vi "Actor Core.vi"(8 "error in":errorcluster, 11 "CS++DeviceGUIActor.lvclass":refnum<class "CS++DeviceGUIActor.lvclass">) -> (0 "Error Out":errorcluster, 3 "Actor out":refnum<class "Actor.lvclass">)   [LabVIEW 2014, in "CS++DeviceGUIActor.lvlib" / "CS++DeviceGUIActor.lvclass"]
doc: "(<B>Filename</B>: Actor Framework.lvlib:Actor.lvclass:Actor Core.vi)\n\nReceives messages to the actor, reacts to them, and initiates any error handling that may shut the actor down.\n\nDescendant classes may override this VI to append parallel tasks for the actor to complete while it handles messages. Overrides use the Call Parent Method node."
uses:
  CS++DeviceGUIActor.lvclass
  <vilib>/ActorFramework/Actor/Actor.lvclass
  CS++BaseActor/CS++BaseActor.lvclass/CS++BaseActor.ctl
  <vilib>/ActorFramework/Actor/Actor.lvclass/Actor.ctl
  <vilib>/ActorFramework/Message Enqueuer/Message Enqueuer.lvclass/Message Enqueuer.ctl
  CS++SVMonitor/CS++SVMonitor.lvclass
  Classes/CS++ProcessVariables/ProcessVariable/PV.lvclass
  CS++DeviceGUIActor Messages/Update PV.lvclass
  CS++PVMonitor Messages/Register PVs Msg/Register PVs Msg.lvclass/Register PVs Msg.ctl
  CS++DeviceGUIActor.lvclass/CS++DeviceGUIActor.ctl
  CS++GUIActor/CS++GUIActor.lvclass/CS++GUIActor.ctl
  Classes/CS++ProcessVariables/ProcessVariable/PV.lvclass/PV.ctl
  Classes/CS++ProcessVariables/ProcessVariable/Read Data.vi
  Classes/CS++ProcessVariables/ProcessVariable/Read Name.vi
  Classes/CS++ProcessVariables/ProcessVariable/Read Timestamp.vi
  <vilib>/ActorFramework/Message Enqueuer/Init from Existing Queue.vi
  <vilib>/ActorFramework/Message Enqueuer/Enqueue.vi
  <vilib>/ActorFramework/Message Priority Queue/Priority Enqueue.vi
  <vilib>/ActorFramework/Stop Msg/Stop Msg.lvclass
  <vilib>/ActorFramework/Message Enqueuer/Message Enqueuer.lvclass
  CS++PVMonitor Messages/Register PVs Msg/Register PVs Msg.lvclass
  Classes/CS++BaseClasses/Factory/CS++Factory.lvclass
  CS++GUIActor/CS++GUIActor.lvclass
  CS++BaseActor/CS++BaseActor.lvclass
panel:
  out "Timestamp":timestamp
  out "Resource Name":string
  out "Self-Test Result Message":string
  out "Self-Test Result Code":i32
  out "Firmware Revision":string
  out "Driver Revision":string
  in  "Stop Button":bool
  out "Associated Actor":string
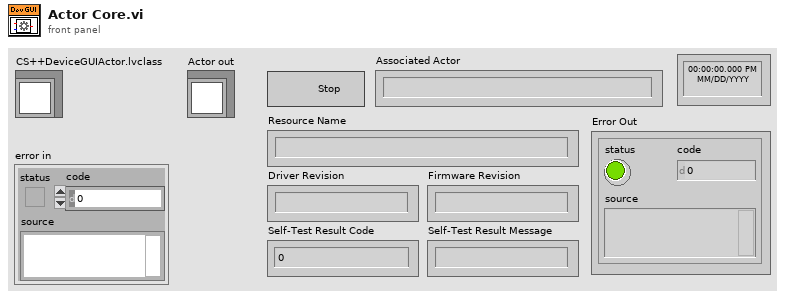
[diagram p1: front panel]
types:
  T1 = enum32{"Invalid", "Standard", "Closed", "Hidden", "Minimized", "Maximized"}
  T2 = cluster{string, "CS++DeviceGUIActor.lvlib:Update PV.lvclass":refnum<class "Update PV.lvclass">}
  T3 = cluster{"Self Enqueuer":refnum<class "Message Enqueuer.lvclass">, cluster{string, "CS++DeviceGUIActor.lvlib:Update PV.lvclass":refnum<class "Update PV.lvclass">}[]}
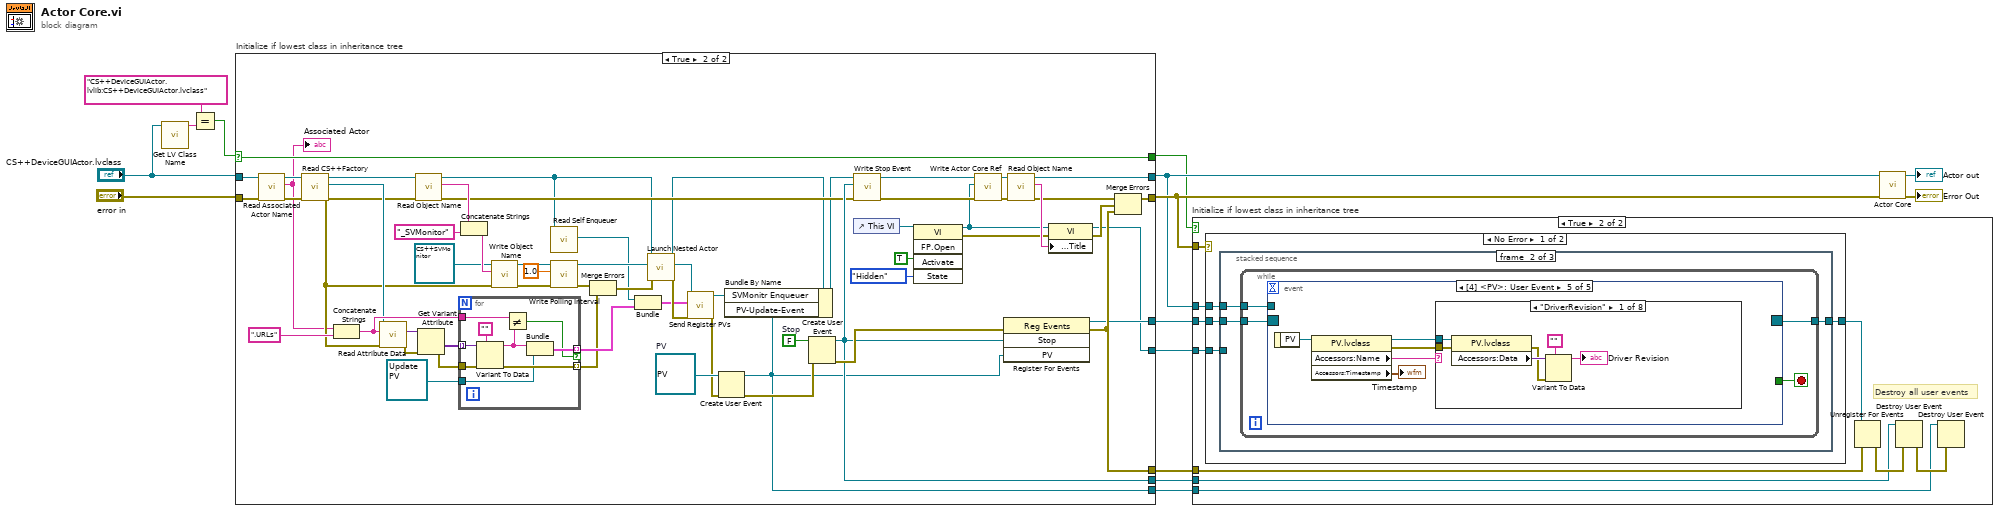
[diagram p0: block diagram]
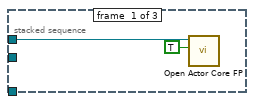
[diagram p4: hidden frame]
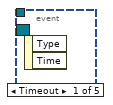
[diagram p5: hidden frame]
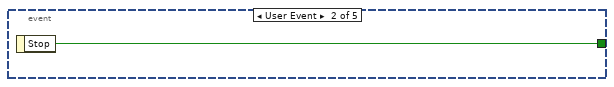
[diagram p6: hidden frame]
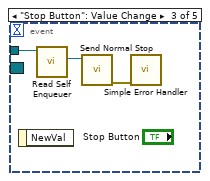
[diagram p7: hidden frame]
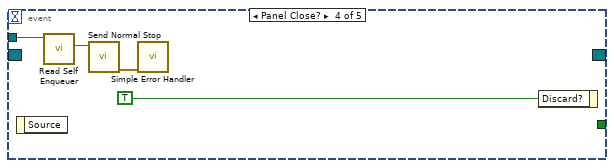
[diagram p8: hidden frame]
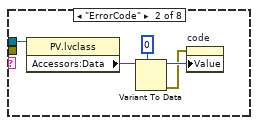
[diagram p9: hidden frame]
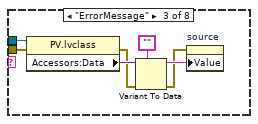
[diagram p10: hidden frame]
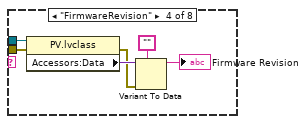
[diagram p11: hidden frame]
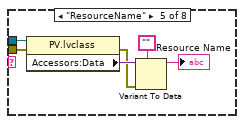
[diagram p12: hidden frame]
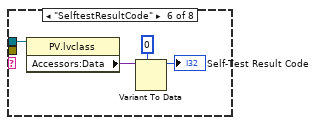
[diagram p13: hidden frame]
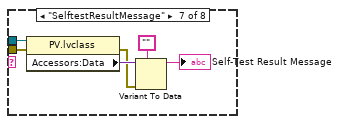
[diagram p14: hidden frame]
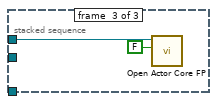
[diagram p16: hidden frame]
diagram:
  n1 = call <vilib>:"Get LV Class Name.vi"("object"="CS++DeviceGUIActor.lvclass") -> ("class name"=w9:string)  [unwired: 9 in, 1 out]
  n2 = Equal?(x="CS++DeviceGUIActor.lvlib:CS++DeviceGUIActor.lvclass" ("class name"), y=w9) -> (x = y?=w3:bool)
  n3 = case "Initialize if lowest class in inheritance tree" shown="True" w3 {
    selector: w3 -> [w16 w61]
    tunnel: [w17 w79] -> w13
    tunnel: "error in" -> [w17 w36]
    tunnel: [w18 w78] -> w11
    tunnel: "CS++DeviceGUIActor.lvclass" -> [w18 w35]
    tunnel: [_ w70] -> w7
    tunnel: [_ w69] -> w6
    tunnel: [_ w59] -> w5
    tunnel: [_ w67] -> w4
    tunnel: [w16 w61] -> w2
    tunnel: [_ w22] -> w1
    frame False {
    }
    frame True {
      w29 = refnum<class "PV.lvclass"> refnum  # PV
      w73 = FALSE  # Stop
      n4 = call "Read Associated Actor Name.vi"("error in (no error)"=w36, "CS++GUIActor in"=w35) -> ("error out"=w34:errorcluster, "Associated Actor Name"=w27:string, "CS++GUIActor out"=w33:refnum<class "CS++DeviceGUIActor.lvclass">)  [unwired: 7 in]
      "Associated Actor" <- w27
      n5 = call "Read CS++Factory.vi"("error in (no error)"=w34, "CS++BaseActor in"=w33) -> ("error out"=w30:errorcluster, "CS++Factory"=w32:refnum<class "CS++Factory.lvclass">, "CS++BaseActor out"=w31:refnum<class "CS++DeviceGUIActor.lvclass">)  [unwired: 7 in]
      n6 = Concatenate Strings(w27, ".URLs" ("string")) -> (w51:string)
      n7 = call-dynamic "Read Attribute Data.vi"("error in (no error)"=w30, "Object Name"=w51, "CS++Factory in"=w32) -> ("error out"=w57:errorcluster, "Attribute Data"=w56:variant)  [unwired: 6 in, 1 out]
      n8 = call "Read Object Name.vi"("error in (no error)"=w30, "CS++BaseActor in"=w31) -> ("error out"=w26:errorcluster, "Object Name"=w44:string, "CS++BaseActor out"=w20:refnum<class "CS++DeviceGUIActor.lvclass">)  [unwired: 7 in]
      n9 = Get Variant Attribute(Variant=w56, error in=w57) -> (values=w50:variant[], error out=w49:errorcluster)  [unwired: 2 in, 2 out]
      n10 = for {
        tunnel: [w88] -> w55 mode=indexing if=w84
        tunnel: w50 -> [w87] mode=indexing
        tunnel: w49 -> [w86]
        tunnel: w51 -> [w85]
        tunnel: [w81] -> w54 mode=indexing
        tunnel: refnum<class "Update PV.lvclass"> refnum ("CS++DeviceGUIActor.lvlib:Update PV.lvclass") -> [w80]
        n11 = Variant To Data(error in=w86, type="", Variant=w87) -> (data=w82:string, error out=w81:errorcluster)
        n12 = Not Equal?(x=w85, y=w82) -> (x != y?=w84:bool)
        n13 = Bundle(w82, "CS++DeviceGUIActor.lvlib:Update PV.lvclass"=w80) -> (w88:T2)  [unwired: 1 in]
      }
      n14 = Concatenate Strings(w44, "_SVMonitor" ("Object Name")) -> (w41:string)
      n15 = call "Write Object Name.vi"("error in (no error)"=w30, "Object Name"=w41, "CS++BaseActor in"=refnum<class "CS++SVMonitor.lvclass"> refnum ("CS++SVMonitor.lvlib:CS++SVMonitor.lvclass")) -> ("error out"=w38:errorcluster, "CS++BaseActor out"=w40:refnum<class "CS++SVMonitor.lvclass">)  [unwired: 7 in]
      n16 = call <vilib>:"Read Self Enqueuer.vi"("Actor"=w20) -> ("Self Enqueuer"=w45:refnum<class "Message Enqueuer.lvclass">)  [unwired: 10 in]
      n17 = call "Write Polling Interval.vi"("error in (no error)"=w38, "Polling Interval"=dbl[unit] 1.0 ("Interval"), "CS++BaseActor in"=w40) -> ("error out"=w52:errorcluster, "CS++BaseActor out"=w58:refnum<class "CS++SVMonitor.lvclass">)  [unwired: 7 in]
      n18 = Merge Errors(w52, w54) -> (w53:errorcluster)
      n19 = Bundle("Self Enqueuer"=w45, w55) -> (w46:T3)  [unwired: 1 in]
      n20 = call <vilib>:"Launch Nested Actor.vi"("error in (no error)"=w53, "Nested Actor"=w58, "Caller Actor in"=w20) -> ("error out"=w47:errorcluster, "Nested Actor's Enqueuer"=w37:refnum<class "Message Enqueuer.lvclass">, "Caller Actor out"=w19:refnum<class "CS++DeviceGUIActor.lvclass">)  [unwired: 6 in]
      n21 = call "Send Register PVs.vi"("error in (no error)"=w47, "Register Info"=w46, "Message Enqueuer"=w37) -> ("error out"=w25:errorcluster, "Message Enqueuer out"=w23:refnum<class "Message Enqueuer.lvclass">)  [unwired: 7 in]
      n22 = Create User Event(user event datatype=w29, error in=w25) -> (user event=w22:refnum<user-event>, error out=w28:errorcluster)
      n23 = Bundle By Name(cluster=w19, "SVMonitr Enqueuer"=w23, "PV-Update-Event"=w22) -> (w24:refnum<class "CS++DeviceGUIActor.lvclass">)
      n24 = Create User Event(user event datatype=w73, error in=w28) -> (user event=w67:refnum<user-event>, error out=w71:errorcluster)
      n25 = call "Write Stop Event.vi"("error in (no error)"=w26, "Stop"=w67, "CS++GUIActor in"=w24) -> ("error out"=w65:errorcluster, "CS++GUIActor out"=w66:refnum<class "CS++DeviceGUIActor.lvclass">)  [unwired: 7 in]
      n26 = control-ref of="This VI"() -> (w77:refnum<vi>)
      n27 = invoke class="VI" method="FP.Open"(reference=w77, "Activate"=TRUE ("Activate?"), "State"=T1."Hidden") -> (reference out=w60:refnum<vi>, error out=w68:errorcluster)  [unwired: 2 in, 3 out]
      n28 = call "Write Actor Core Ref.vi"("error in (no error)"=w65, "Actor Core Ref"=w60, "CS++BaseActor in"=w66) -> ("error out"=w64:errorcluster, "CS++BaseActor out"=w63:refnum<class "CS++DeviceGUIActor.lvclass">)  [unwired: 7 in]
      n29 = register-events(error in=w71, w67, w22) -> (reference out=w69:refnum<event-registration>, error out=w70:errorcluster)  [unwired: 1 in]
      n30 = call "Read Object Name.vi"("error in (no error)"=w64, "CS++BaseActor in"=w63) -> ("error out"=w62:errorcluster, "Object Name"=w74:string, "CS++BaseActor out"=w78:refnum<class "CS++DeviceGUIActor.lvclass">)  [unwired: 7 in]
      n31 = property class="VI"(reference=w60, error in=w68, "Front Panel.Title"=w74) -> (reference out=w59:refnum<vi>, error out=w72:errorcluster)
      n32 = Merge Errors(w62, w72, w70) -> (w79:errorcluster)
    }
  }
  n33 = case "Initialize if lowest class in inheritance tree" shown="True" w2 {
    tunnel: w13 -> [_ w98]
    tunnel: w11 -> [_ w97]
    tunnel: w7 -> [_ w95]
    tunnel: w6 -> [_ w94]
    tunnel: w5 -> [_ w92]
    tunnel: w4 -> [_ w91]
    tunnel: w1 -> [_ w89]
    frame False {
    }
    frame True {
      # "Destroy all user events"
      n34 = case shown="No Error" w98 {
        tunnel: w97 -> [w102 _]
        tunnel: w94 -> [w101 w167]
        tunnel: [w100 w167] -> w93
        tunnel: w92 -> [w99 _]
        frame No Error {
          n35 = stacked-sequence {
            tunnel: w102 -> [w104 w106 w166]
            tunnel: w101 -> [_ w107 _]
            tunnel: [_ w105 _] -> w100
            tunnel: w99 -> [_ _ _]
            frame #0 {
              n36 = call "Open Actor Core FP.vi"("Open FP (F)"=TRUE, "CS++BaseActor in"=w104) -> ()  [unwired: 8 in, 2 out]
            }
            frame #1 {
              n37 = while {
                tunnel: w107 -> [w111]
                tunnel: w106 -> [w110]
                tunnel: [w108] -> w105
                stop <- w109 stop-if-true
                n38 = event shown="[4] <PV>: User Event" {
                  selector: w111 -> [_ _ _ _ _]
                  dyn-events: [_ _ _ _ _] -> w108
                  timeout: _ -> [_ _ _ _ _]
                  tunnel: w110 -> [_ _ w115 w116 _]
                  tunnel: [_ w112 _ _ _] -> w109
                  event Timeout {
                    n39 = event-data() -> ()  [unwired: 1 in, 2 out]
                  }
                  event User Event {
                    n40 = event-data() -> ("Stop"=w112:bool)  [unwired: 1 in]
                  }
                  event "Stop Button": Value Change {
                    n41 = event-data() -> ()  [unwired: 1 in, 1 out]
                    n42 = call <vilib>:"Read Self Enqueuer.vi"("Actor"=w115) -> ("Self Enqueuer"=w114:refnum<class "Message Enqueuer.lvclass">)  [unwired: 10 in]
                    n43 = call <vilib>:"Send Normal Stop.vi"("Message Enqueuer"=w114) -> ("error out"=w113:errorcluster)  [unwired: 10 in]
                    n44 = call <vilib>:"Simple Error Handler.vi"("error in (no error)"=w113) -> ()  [unwired: 4 in, 5 out]
                  }
                  event Panel Close? {
                    n45 = event-data() -> ()  [unwired: 1 in, 1 out]
                    n46 = call <vilib>:"Read Self Enqueuer.vi"("Actor"=w116) -> ("Self Enqueuer"=w118:refnum<class "Message Enqueuer.lvclass">)  [unwired: 10 in]
                    n47 = call <vilib>:"Send Normal Stop.vi"("Message Enqueuer"=w118) -> ("error out"=w117:errorcluster)  [unwired: 10 in]
                    n48 = call <vilib>:"Simple Error Handler.vi"("error in (no error)"=w117) -> ()  [unwired: 4 in, 5 out]
                    n49 = event-data("Discard?"=TRUE) -> ()  [unwired: 1 in, 1 out]
                  }
                  event User Event {
                    n50 = event-data() -> ("PV"=w124:refnum<class "PV.lvclass">)  [unwired: 1 in]
                    n51 = property class="PV.lvclass"(reference=w124) -> (reference out=w123:refnum<class "PV.lvclass">, error out=w122:errorcluster, "Accessors:Name"=w120:string, "Accessors:Timestamp"=→"Timestamp":timestamp)  [unwired: 1 in]
                    n52 = case shown="\"DriverRevision\"" w120 {
                      tunnel: w123 -> [w128 w133 w140 w146 w152 w156 w162 _]
                      tunnel: w122 -> [w127 _ w139 w145 w151 _ w161 _]
                      frame "DriverRevision" {
                        n53 = property class="PV.lvclass"(reference=w128, error in=w127) -> (error out=w126:errorcluster, "Accessors:Data"=w129:variant)  [unwired: 1 out]
                        n54 = Variant To Data(error in=w126, type="", Variant=w129) -> (data=→"Driver Revision":string)  [unwired: 1 out]
                      }
                      frame "ErrorCode" {
                        n55 = property class="PV.lvclass"(reference=w133) -> ("Accessors:Data"=w134:variant)  [unwired: 1 in, 2 out]
                        n56 = Variant To Data(type=0, Variant=w134) -> (data=w132:i32, error out=w131:errorcluster)  [unwired: 1 in]
                        n57 = property on="code" class="DigNum (strict)"(error in=w131, "Value"=w132) -> ()  [unwired: 1 in, 2 out]
                      }
                      frame "ErrorMessage" {
                        n58 = property class="PV.lvclass"(reference=w140, error in=w139) -> (error out=w138:errorcluster, "Accessors:Data"=w141:variant)  [unwired: 1 out]
                        n59 = Variant To Data(error in=w138, type="", Variant=w141) -> (data=w137:string, error out=w136:errorcluster)
                        n60 = property on="source" class="Str"(error in=w136, "Value"=w137) -> ()  [unwired: 1 in, 2 out]
                      }
                      frame "FirmwareRevision" {
                        n61 = property class="PV.lvclass"(reference=w146, error in=w145) -> (error out=w144:errorcluster, "Accessors:Data"=w147:variant)  [unwired: 1 out]
                        n62 = Variant To Data(error in=w144, type="", Variant=w147) -> (data=→"Firmware Revision":string)  [unwired: 1 out]
                      }
                      frame "ResourceName" {
                        n63 = property class="PV.lvclass"(reference=w152, error in=w151) -> (error out=w150:errorcluster, "Accessors:Data"=w153:variant)  [unwired: 1 out]
                        n64 = Variant To Data(error in=w150, type="", Variant=w153) -> (data=→"Resource Name":string)  [unwired: 1 out]
                      }
                      frame "SelftestResultCode" {
                        n65 = property class="PV.lvclass"(reference=w156) -> ("Accessors:Data"=w157:variant)  [unwired: 1 in, 2 out]
                        n66 = Variant To Data(type=0, Variant=w157) -> (data=→"Self-Test Result Code":i32)  [unwired: 1 in, 1 out]
                      }
                      frame "SelftestResultMessage" {
                        n67 = property class="PV.lvclass"(reference=w162, error in=w161) -> (error out=w160:errorcluster, "Accessors:Data"=w163:variant)  [unwired: 1 out]
                        n68 = Variant To Data(error in=w160, type="", Variant=w163) -> (data=→"Self-Test Result Message":string)  [unwired: 1 out]
                      }
                      frame Default {
                      }
                    }
                  }
                }
              }
            }
            frame #2 {
              n69 = call "Open Actor Core FP.vi"("Open FP (F)"=FALSE, "CS++BaseActor in"=w166) -> ()  [unwired: 8 in, 2 out]
            }
          }
        }
        frame Error {
        }
      }
      n70 = Unregister For Events(event registration refnum=w93, error in=w95) -> (error out=w96:errorcluster)
      n71 = Destroy User Event(user event=w91, error in=w96) -> (error out=w90:errorcluster)
      n72 = Destroy User Event(user event=w89, error in=w90) -> ()  [unwired: 1 out]
    }
  }
  n73 = call-parent "Actor Core.vi"("error in"=w13, "CS++GUIActor in"=w11) -> ("error out"=→"Error Out":errorcluster, "Actor out"=→"Actor out":refnum<class "Actor.lvclass">)  [unwired: 8 in]
